vi "CheckState.vi"(8 "Error In":errorcluster, 10 "Module No.":i16, 11 "DLL Path":path) -> (0 "Error Out":errorcluster, 1 "SPC_StateCluster":T1, 2 "Module No.":i16, 3 "DLL Path":path, 4 "State Value":i16)   [LabVIEW 2023]
doc: "This VI is a wrapper for the SPC_test_state.vi and interprets the 'State Value'-flags as a Boolean cluster for convenience.\n<b>Note:</b> SPC_read_state is clearing some flags directly. Take care when using in different threats.\n\n<b>Note:</b> This VI is set to execute as preallocated clone to improve performance when run in parallel loops for multi module setups.\n\ninfo@becker-hickl.com"
uses:
  SPC_Controls/StateCluster.ctl
panel:
  # "Note: \nSPC_read_state is clearing some flags directly"
  # "See Tip-Strip for details"
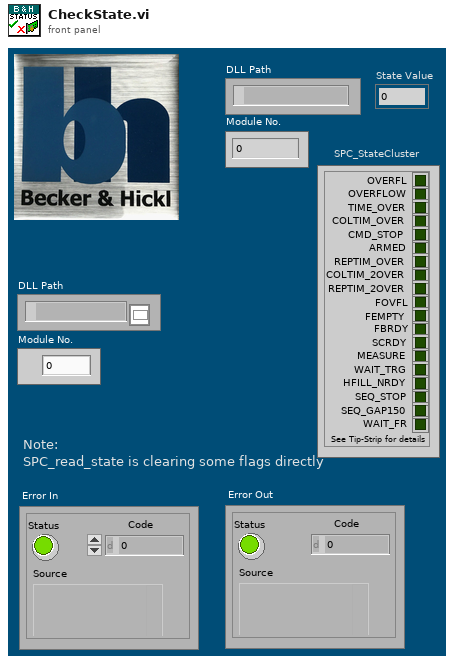
[diagram p1: front panel]
types:
  T1 = typedef "StateCluster.ctl" = cluster{"OVERFL":bool, "OVERFLOW":bool, "TIME_OVER":bool, "COLTIM_OVER":bool, "CMD_STOP":bool, "ARMED":bool, "REPTIM_OVER":bool, "COLTIM_2OVER":bool, "REPTIM_2OVER":bool, "FOVFL":bool, "FEMPTY":bool, "FBRDY":bool, "SCRDY":bool, "MEASURE":bool, "WAIT_TRG":bool, "HFILL_NRDY":bool, "SEQ_STOP":bool, "SEQ_GAP150":bool, "WAIT_FR":bool}
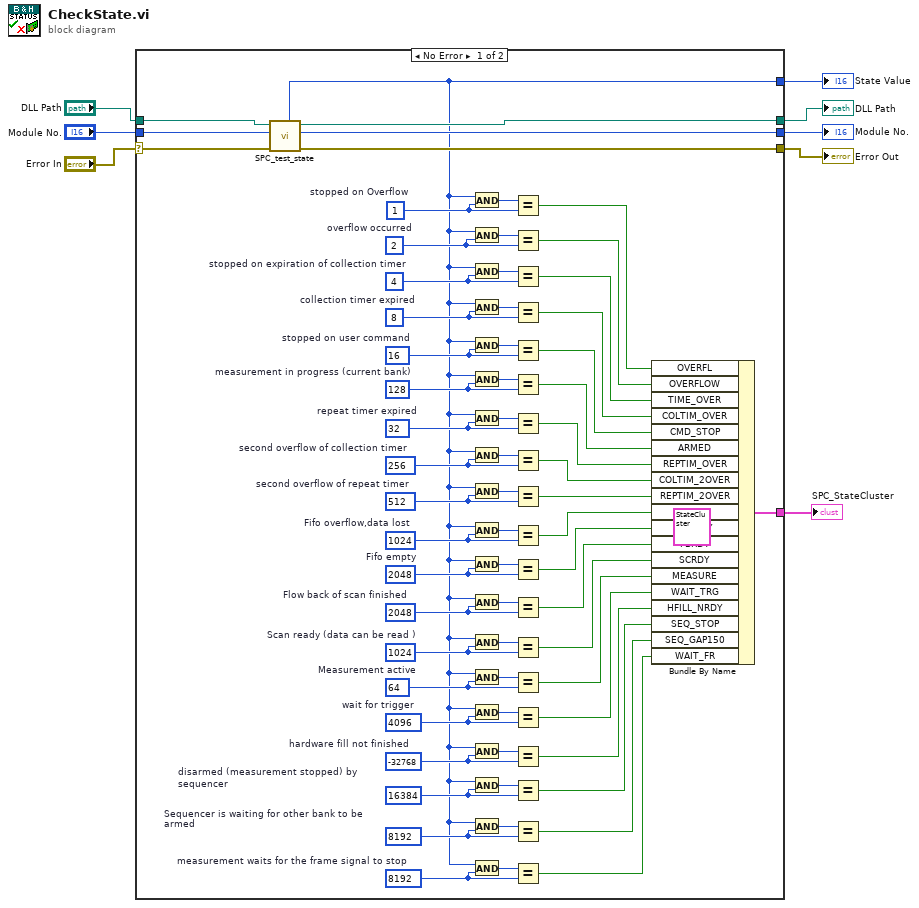
[diagram p0: block diagram]
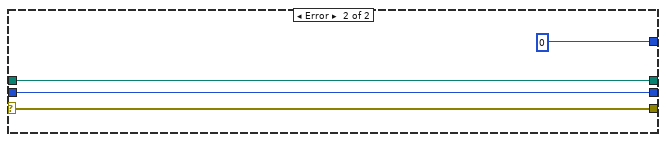
[diagram p2: hidden frame]
diagram:
  n1 = case shown="No Error" "Error In" {
    selector: "Error In" -> [w66 w78]
    tunnel: "DLL Path" -> [w71 w76]
    tunnel: "Module No." -> [w70 w77]
    tunnel: [w69 w77] -> w6
    tunnel: [w68 w76] -> w5
    tunnel: [w67 w78] -> w4
    tunnel: [w9 i16 0] -> w1
    tunnel: [w10 _] -> w2
    frame No Error {
      w12 = i16 8192  # measurement waits for the frame signal to stop
      w16 = i16 8192  # Sequencer is waiting for other bank to be armed
      w18 = i16 16384  # disarmed (measurement stopped) by sequencer
      w22 = i16 -32768  # hardware fill not finished
      w24 = i16 4096  # wait for trigger
      w28 = i16 64  # Measurement active
      w30 = i16 1024  # Scan ready (data can be read )
      w34 = i16 2048  # Flow back of scan finished
      w36 = i16 2048  # Fifo empty
      w40 = i16 1024  # Fifo overflow,data lost
      w42 = i16 512  # second overflow of repeat timer
      w46 = i16 256  # second overflow of collection timer
      w48 = i16 32  # repeat timer expired
      w54 = i16 16  # stopped on user command
      w60 = i16 128  # measurement in progress (current bank)
      w61 = i16 8  # collection timer expired
      w64 = i16 4  # stopped on expiration of collection timer
      w65 = i16 2  # overflow occurred
      w74 = i16 1  # stopped on Overflow
      n2 = call "SPC_test_state.vi"("Error In"=w66, "Module No"=w70, "DLL Path"=w71) -> ("Error Out"=w67:errorcluster, "Module No"=w69:i16, "DLL Path"=w68:path, "State Value"=w9:i16)  [unwired: 5 in]
      n3 = And(x=w9, y=w74) -> (x .and. y?=w73:i16)
      n4 = And(x=w9, y=w65) -> (x .and. y?=w72:i16)
      n5 = And(x=w9, y=w64) -> (x .and. y?=w63:i16)
      n6 = And(x=w9, y=w61) -> (x .and. y?=w62:i16)
      n7 = And(x=w9, y=w54) -> (x .and. y?=w53:i16)
      n8 = And(x=w9, y=w60) -> (x .and. y?=w59:i16)
      n9 = And(x=w9, y=w48) -> (x .and. y?=w49:i16)
      n10 = And(x=w9, y=w46) -> (x .and. y?=w45:i16)
      n11 = And(x=w9, y=w42) -> (x .and. y?=w43:i16)
      n12 = And(x=w9, y=w40) -> (x .and. y?=w39:i16)
      n13 = And(x=w9, y=w36) -> (x .and. y?=w37:i16)
      n14 = And(x=w9, y=w34) -> (x .and. y?=w33:i16)
      n15 = And(x=w9, y=w30) -> (x .and. y?=w31:i16)
      n16 = And(x=w9, y=w28) -> (x .and. y?=w27:i16)
      n17 = And(x=w9, y=w24) -> (x .and. y?=w25:i16)
      n18 = And(x=w9, y=w22) -> (x .and. y?=w21:i16)
      n19 = And(x=w9, y=w18) -> (x .and. y?=w19:i16)
      n20 = And(x=w9, y=w16) -> (x .and. y?=w15:i16)
      n21 = And(x=w9, y=w12) -> (x .and. y?=w13:i16)
      n22 = Equal?(x=w73, y=w74) -> (x = y?=w57:bool)
      n23 = Equal?(x=w72, y=w65) -> (x = y?=w56:bool)
      n24 = Equal?(x=w63, y=w64) -> (x = y?=w55:bool)
      n25 = Equal?(x=w62, y=w61) -> (x = y?=w51:bool)
      n26 = Equal?(x=w53, y=w54) -> (x = y?=w52:bool)
      n27 = Equal?(x=w59, y=w60) -> (x = y?=w50:bool)
      n28 = Equal?(x=w49, y=w48) -> (x = y?=w47:bool)
      n29 = Equal?(x=w45, y=w46) -> (x = y?=w44:bool)
      n30 = Equal?(x=w43, y=w42) -> (x = y?=w41:bool)
      n31 = Equal?(x=w39, y=w40) -> (x = y?=w38:bool)
      n32 = Equal?(x=w37, y=w36) -> (x = y?=w35:bool)
      n33 = Equal?(x=w33, y=w34) -> (x = y?=w32:bool)
      n34 = Equal?(x=w31, y=w30) -> (x = y?=w29:bool)
      n35 = Equal?(x=w27, y=w28) -> (x = y?=w26:bool)
      n36 = Equal?(x=w25, y=w24) -> (x = y?=w23:bool)
      n37 = Equal?(x=w21, y=w22) -> (x = y?=w20:bool)
      n38 = Equal?(x=w19, y=w18) -> (x = y?=w17:bool)
      n39 = Equal?(x=w15, y=w16) -> (x = y?=w14:bool)
      n40 = Equal?(x=w13, y=w12) -> (x = y?=w11:bool)
      n41 = Bundle By Name(cluster=T1 {"OVERFL"=FALSE, "OVERFLOW"=TRUE, "TIME_OVER"=TRUE, "COLTIM_OVER"=TRUE, "CMD_STOP"=FALSE, "ARMED"=TRUE, "REPTIM_OVER"=FALSE, "COLTIM_2OVER"=TRUE, "REPTIM_2OVER"=FALSE, "FOVFL"=TRUE, "FEMPTY"=FALSE, "FBRDY"=TRUE, "SCRDY"=FALSE, "MEASURE"=TRUE, "WAIT_TRG"=TRUE, "HFILL_NRDY"=TRUE, "SEQ_STOP"=TRUE, "SEQ_GAP150"=FALSE, "WAIT_FR"=TRUE} ("SPC_StateCluster"), "OVERFL"=w57, "OVERFLOW"=w56, "TIME_OVER"=w55, "COLTIM_OVER"=w51, "CMD_STOP"=w52, "ARMED"=w50, "REPTIM_OVER"=w47, "COLTIM_2OVER"=w44, "REPTIM_2OVER"=w41, "FOVFL"=w38, "FEMPTY"=w35, "FBRDY"=w32, "SCRDY"=w29, "MEASURE"=w26, "WAIT_TRG"=w23, "HFILL_NRDY"=w20, "SEQ_STOP"=w17, "SEQ_GAP150"=w14, "WAIT_FR"=w11) -> (w10:T1)
    }
    frame Error {
    }
  }
  "DLL Path" <- w5
  "Module No." <- w6
  "Error Out" <- w4
  "SPC_StateCluster" <- w2
  "State Value" <- w1
